vi "Cancel State Machine - Pickup.vi"   [LabVIEW 2013]
uses:
  typedefs/State Machine/subStates.ctl
  typedefs/fg_typedef.ctl
  typedefs/DevRef Type.ctl
panel:
  # "A State Machine to Handle Canceling Pickup"
types:
  T1 = typedef "subStates.ctl" = enum16{"null", "wait", "driver control", "auto", "manual override", "hold position", "rotate", "pickup", "pass", "recover pass", "load", "goto shoot", "shoot high goal", "shoot low goal", "cancel arm", "cancel shooter", "end", "test"}
  T2 = typedef "DevRef Type.ctl" = enum16{"Shooter Solenoid", "Latch Solenoid", "Right Up Sensor", "Right Down Sensor", "Hold Sensor", "2 Ball Switch", "Arm Encoder"}
  T3 = typedef "fg_typedef.ctl" = enum16{"Get", "Set"}
  T4 = typedef "WPI_EncoderDevRef.ctl" = cluster{"DevStatus":errorcluster, "EncoderIndex":T5, "CounterIndex":T6, "DistancePerCount":dbl, "Decoding Type":T7}
  T5 = typedef "FPGA_EncoderIdx.ctl" = enum8{"Enc 0", "Enc 1", "Enc 2", "Enc 3", "Invalid"}
  T6 = typedef "FPGA_CounterCtrSystemIndex.ctl" = enum8{"Ctr 0", "Ctr 1", "Ctr 2", "Ctr 3", "Ctr 4", "Ctr 5", "Ctr 6", "Ctr 7", "Invalid"}
  T7 = typedef "WPI_EncoderType.ctl" = enum16{"1x", "2x", "4x"}
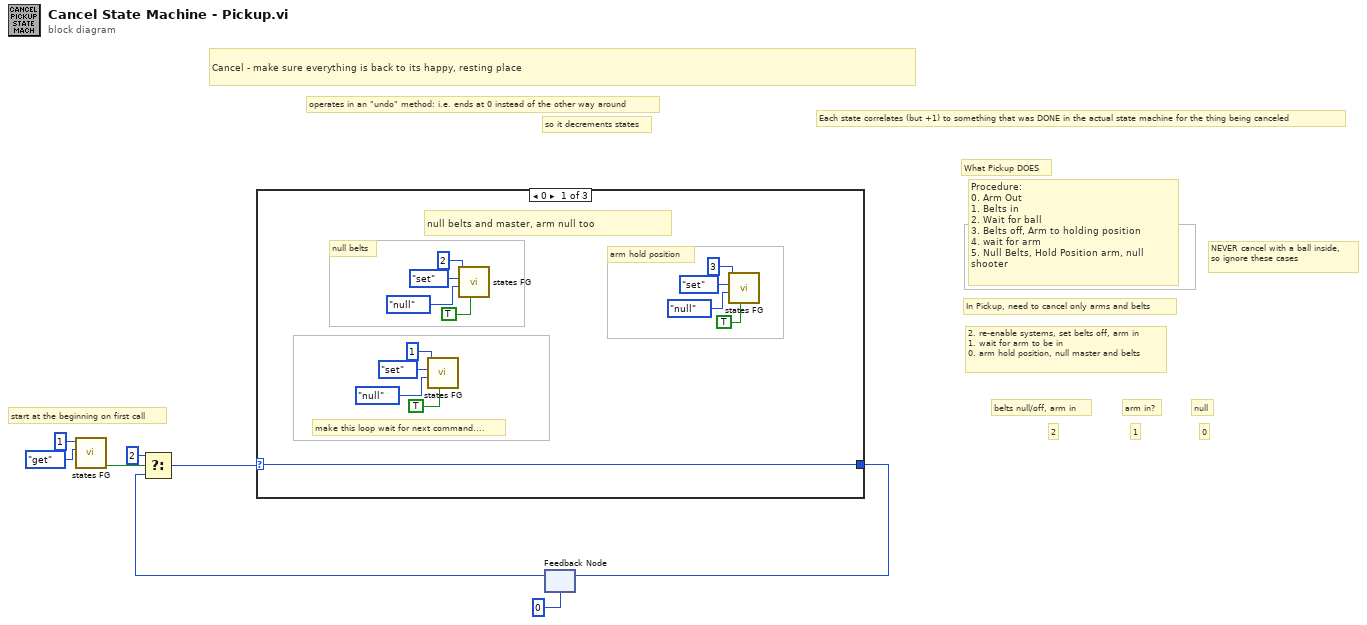
[diagram p0: block diagram]
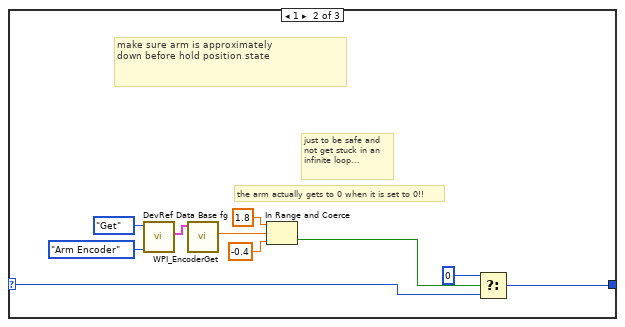
[diagram p2: hidden frame]
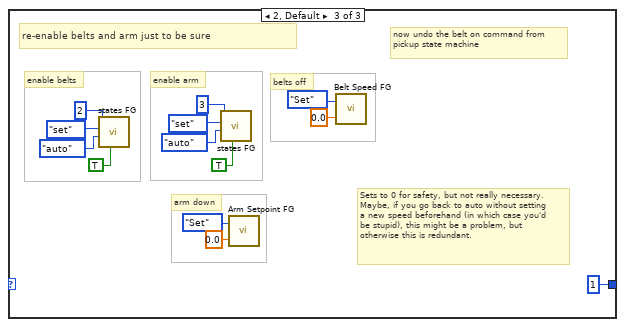
[diagram p3: hidden frame]
diagram:
  # "0"
  # "null"
  # "1"
  # "2"
  # "arm in?"
  # "belts null/off, arm in"
  # "NEVER cancel with a ball inside,\nso ignore these cases"
  # "so it decrements states"
  # "What Pickup DOES"
  # "Each state correlates (but +1) to something that was DONE in the actual state machine for the thing being canceled"
  # "operates in an \"undo\" method: i.e. ends at 0 instead of the other way around"
  # "2. re-enable systems, set belts off, arm in\n1. wait for arm to be in\n0. arm hold position, null master and belts"
  # "In Pickup, need to cancel only arms and belts"
  # "start at the beginning on first call"
  # "Cancel - make sure everything is back to its happy, resting place"
  # "Procedure: \n0. Arm Out\n1. Belts in\n2. Wait for ball\n3. Belts off, Arm to holding position\n4. wait for arm\n5. Null Belts, Hold Position arm, null shooter"
  n1 = call "states FG.vi"("menu (get)"=enum16{"set", "get"}."get", "Loop ID"=1) -> ("first call?"=w8:bool)  [unwired: 6 in, 3 out]
  n2 = feedback #1(u8 0) -> (w3:u8)
  n3 = Select(t=u8 2, s=w8, f=w3) -> (s? t:f=w5:u8)
  n4 = case shown="0" w5 {
    selector: w5 -> [w21 w27 _]
    tunnel: [w21 w26 u8 1 ("t")] -> w2
    frame 0 {
      # "null belts and master, arm null too"
      # "make this loop wait for next command...."
      # "arm hold position"
      # "null belts"
      n5 = call "states FG.vi"("exit in"=TRUE, "subState in"=subStates."null", "menu (get)"=enum16{"set", "get"}."set", "Loop ID"=1) -> ()  [unwired: 4 in, 4 out]
      n6 = call "states FG.vi"("exit in"=TRUE, "subState in"=subStates."null", "menu (get)"=enum16{"set", "get"}."set", "Loop ID"=2) -> ()  [unwired: 4 in, 4 out]
      n7 = call "states FG.vi"("exit in"=TRUE, "subState in"=subStates."null", "menu (get)"=enum16{"set", "get"}."set", "Loop ID"=3) -> ()  [unwired: 4 in, 4 out]
    }
    frame 1 {
      # "just to be safe and\nnot get stuck in an \ninfinite loop..."
      # "the arm actually gets to 0 when it is set to 0!!"
      # "make sure arm is approximately\ndown before hold position state"
      n8 = call "DevRef Data Base fg.vi"("DevRef to Get"=DevRef_Type."Arm Encoder", "Menu"=fg_typedef."Get") -> ("Selected Encoder"=w31:T4)  [unwired: 2 in, 5 out]
      n9 = call <vilib>:"WPI_EncoderGet.vi"("EncoderDevRef"=w31) -> ("Distance"=w30:dbl)  [unwired: 5 in, 5 out]
      n10 = In Range and Coerce(upper limit=1.8, x=w30, lower limit=-0.4 ("upper limit")) -> (In Range?=w24:bool)  [unwired: 1 out]
      n11 = Select(t=u8 0, s=w24, f=w27) -> (s? t:f=w26:u8)
    }
    frame 2, Default {
      # "arm down"
      # "Sets to 0 for safety, but not really necessary.\nMaybe, if you go back to auto without setting\na new speed beforehand (in which case you'd\nbe stupid), this might be a problem, but\notherwise this is redundant."
      # "now undo the belt on command from\npickup state machine"
      # "belts off"
      # "re-enable belts and arm just to be sure"
      # "enable arm"
      # "enable belts"
      n12 = call "states FG.vi"("exit in"=TRUE, "subState in"=subStates."auto", "menu (get)"=enum16{"set", "get"}."set", "Loop ID"=2) -> ()  [unwired: 4 in, 4 out]
      n13 = call "states FG.vi"("exit in"=TRUE, "subState in"=subStates."auto", "menu (get)"=enum16{"set", "get"}."set", "Loop ID"=3) -> ()  [unwired: 4 in, 4 out]
      n14 = call "Arm Setpoint FG.vi"("Setpoint In"=0.0, "Menu"=fg_typedef."Set") -> ()  [unwired: 1 out]
      n15 = call "Belt Speed FG.vi"("Speed In"=0.0 ("Setpoint In"), "Menu"=fg_typedef."Set") -> ()  [unwired: 1 out]
    }
  }
  n16 = feedback-in #1(w2) -> ()
